vi "Peg-in-hole 2015-03-09 data.vi"() -> ()   [LabVIEW 2013]
uses:
  <vilib>/Analysis/baseanly.llb/Mean (DBL).vi
  <vilib>/Analysis/NI_AALBase.lvlib
  <vilib>/Analysis/NI_AALPro.lvlib
  <vilib>/gmath/NI_Gmath.lvlib
panel:
  in  "Times":dbl[](array[numeric])=[27.75, 28.05, 27.9, 17.75, 143.25, 110.6, 42.95, 17.2, 41.6, 16.8, 27.95, 65.9, 30.25, 18.5, 17.5, 48.1, 62.35, 17.55, 52.75, 322.0, 27.9, 27.45, 27.2, 18.0, 17.4, 27.95, 51.2, 17.55, 40.2, 171.4, 28.25, 27.85, 27.35, 17.85, 16.95, 39.3, 38.75, 17.35, 29.45, 17.2, 27.8, 28.15, 142.2, 63.6, 17.65, 89.651, 28.5, 17.55, 29.0, 17.15, 17.65, 28.45, 28.45, 42.9, 16.75, 38.55, 39.45, 17.8, 208.85, 49.9, 17.25, 37.75, 69.85, 29.9, 17.3, 17.5, 19.1, 80.35, 31.499, 80.55, 17.45, 17.65, 27.95, 40.65, 17.25, 70.15, 28.8, 17.4, 18.4, 17.55, 16.95, 50.4, 27.15, 52.5, 16.85, 17.6, 39.6, 17.35, 18.35, 17.75, 58.15, 71.55, 27.65, 107.75, 16.95, 28.75, 28.7, 17.5, 128.9, 59.35]
  in  "y":dbl
  out "correlation coefficient r":dbl
  out "offset":dbl
  out "power":dbl
  out "amplitude":dbl
  out "XY Graph":cluster{cluster{dbl, "mean":dbl}[]}[](graph)
  # "Data from central taught point"
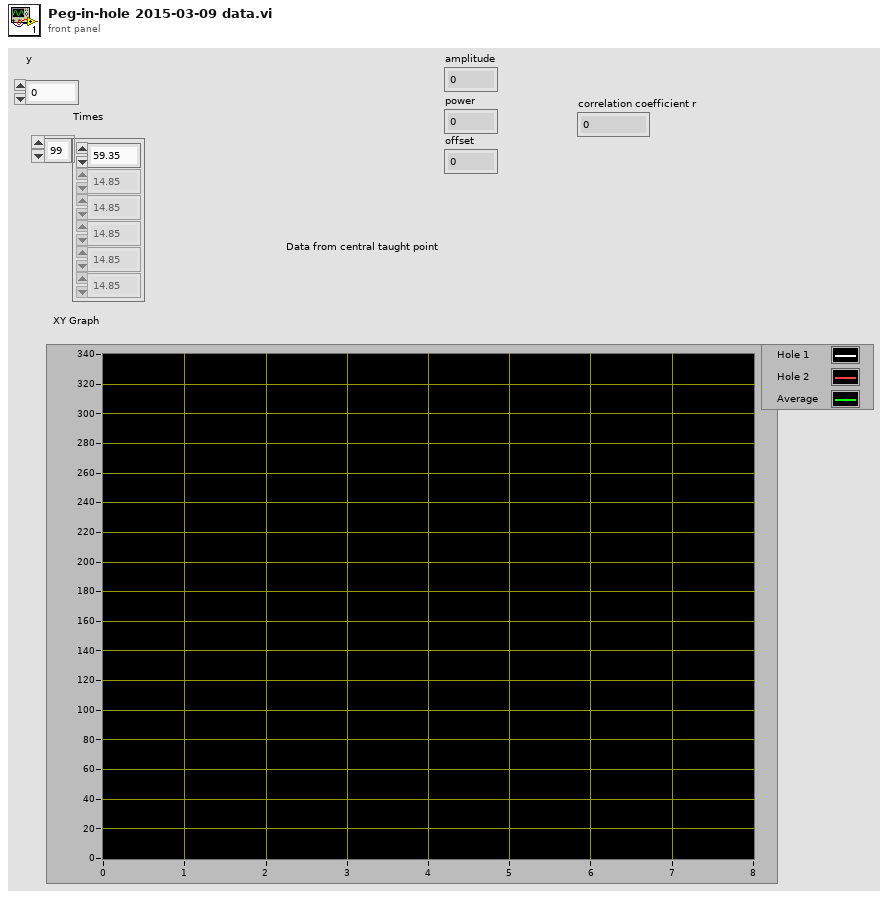
[diagram p1: front panel]
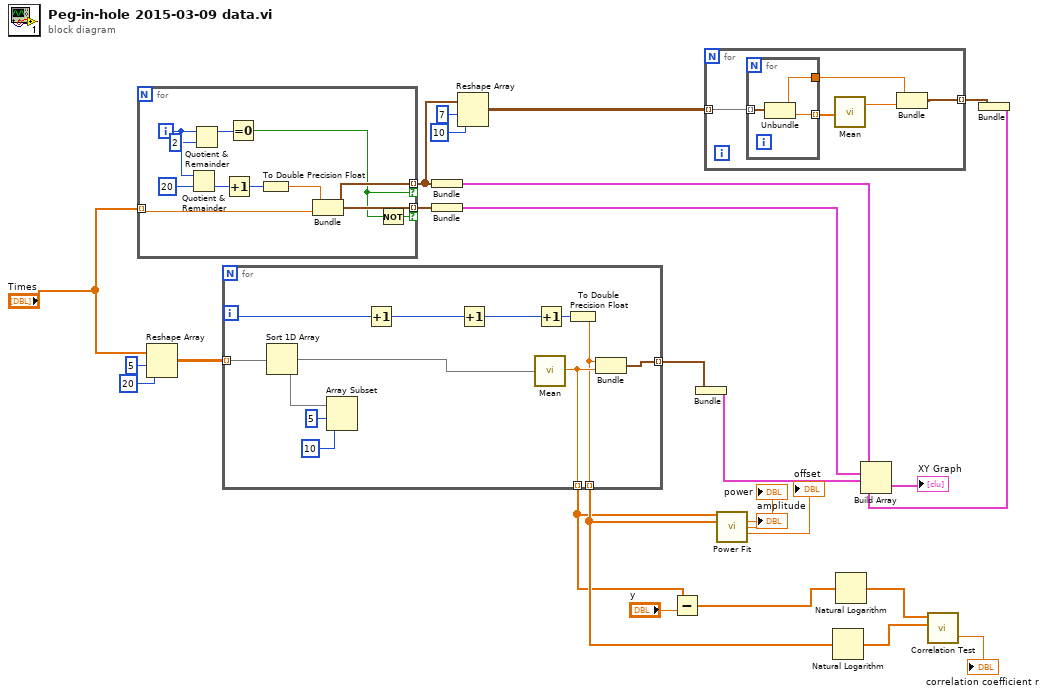
[diagram p0: block diagram]
diagram:
  n1 = for {
    tunnel: "Times" -> [w27] mode=indexing
    tunnel: [w30] -> w22 mode=indexing if=w28
    tunnel: [w30] -> w4 mode=indexing if=w29
    i -> [w33]
    n2 = Quotient & Remainder(x=w33, y=20) -> (floor(x/y)=w36:i32)  [unwired: 1 out]
    n3 = Quotient & Remainder(x=w33, y=2) -> (x-y*floor(x/y)=w31:i32)  [unwired: 1 out]
    n4 = Increment(x=w36) -> (x+1=w35:i32)
    n5 = Equal To 0?(x=w31) -> (x = 0?=w29:bool)
    n6 = To Double Precision Float(number=w35) -> (double precision float=w34:dbl)
    n7 = Bundle(w34, w27) -> (w30:cluster{dbl, dbl})  [unwired: 1 in]
    n8 = Not(x=w29) -> (.not. x?=w28:bool)
  }
  n9 = Reshape Array("Times", 5 ("dimension size"), 20 ("dimension size")) -> (w24:dbl[][])
  n10 = for {
    tunnel: w24 -> [w43] mode=indexing
    tunnel: [w46] -> w23 mode=indexing
    tunnel: [w45] -> w10 mode=indexing
    tunnel: [w44] -> w14 mode=indexing
    i -> [w48]
    n11 = Sort 1D Array(array=w43) -> (sorted array=w40:dbl[])
    n12 = Array Subset(array=w40, index=5, length=10) -> ()  [unwired: 1 out]
    n13 = Increment(x=w48) -> (x+1=w38:i32)
    n14 = Increment(x=w38) -> (x+1=w39:i32)
    n15 = call-poly <vilib>:"Mean.vi"("X"=w40) -> ("mean"=w45:dbl)  [unwired: 1 out]
    n16 = Increment(x=w39) -> (x+1=w47:i32)
    n17 = To Double Precision Float(number=w47) -> (double precision float=w44:dbl)
    n18 = Bundle(w44, "mean"=w45) -> (w46:cluster{dbl, "mean":dbl})  [unwired: 1 in]
  }
  n19 = Bundle(w4) -> (w7:cluster{cluster{dbl, dbl}[]})  [unwired: 1 in]
  n20 = Bundle(w22) -> (w20:cluster{cluster{dbl, dbl}[]})  [unwired: 1 in]
  n21 = Reshape Array(w4, 7 ("dimension size"), 10 ("dimension size")) -> (w3:cluster{dbl, dbl}[][])
  n22 = Subtract(x=w10, y="y") -> (x-y=w9:dbl[])
  n23 = Bundle(w23) -> (w19:cluster{cluster{dbl, "mean":dbl}[]})  [unwired: 1 in]
  n24 = for {
    tunnel: w3 -> [w53] mode=indexing
    tunnel: [w49] -> w2 mode=indexing
    n25 = for {
      tunnel: w53 -> [w56] mode=indexing
      tunnel: [w55] -> w52 mode=indexing
      tunnel: [w54] -> w51
      n26 = Unbundle(w56) -> (w54:dbl, w55:dbl)
    }
    n27 = call-poly <vilib>:"Mean.vi"("X"=w52) -> ("mean"=w50:dbl)  [unwired: 1 out]
    n28 = Bundle(w51, "mean"=w50) -> (w49:cluster{dbl, "mean":dbl})  [unwired: 1 in]
  }
  n29 = call <vilib>:"Power Fit.vi"("Y"=w10, "X"=w14) -> ("amplitude"=→"amplitude":dbl, "power"=→"power":dbl, "offset"=→"offset":dbl)  [unwired: 8 in, 3 out]
  n30 = Natural Logarithm(1:w14) -> (0:w12:dbl[])
  n31 = Natural Logarithm(1:w9) -> (0:w13:dbl[])
  n32 = call <vilib>:"Correlation Test.vi"("sample set y"=w12, "sample set x"=w13) -> ("correlation coefficient r"=→"correlation coefficient r":dbl)  [unwired: 5 in, 4 out]
  n33 = Bundle(w2) -> (w1:cluster{cluster{dbl, "mean":dbl}[]})  [unwired: 1 in]
  n34 = Build Array(w7, w20, w19, w1) -> (→"XY Graph":cluster{cluster{dbl, "mean":dbl}[]}[])
